vi "DAQAdvance.vi"() -> ()   [LabVIEW 2018]
uses:
  <vilib>/DAQmx/read.llb/DAQmx Read (Analog DBL 1Chan 1Samp).vi
  <vilib>/DAQmx/write.llb/DAQmx Write (Analog DBL 1Chan 1Samp).vi
  <vilib>/DAQmx/miscellaneous.llb/DAQmx Fill In Error Info.vi
panel:
  out "Waveform Chart":cluster{dbl, "data":dbl}(graph)
  in  "y":i32
  in  "stop":bool
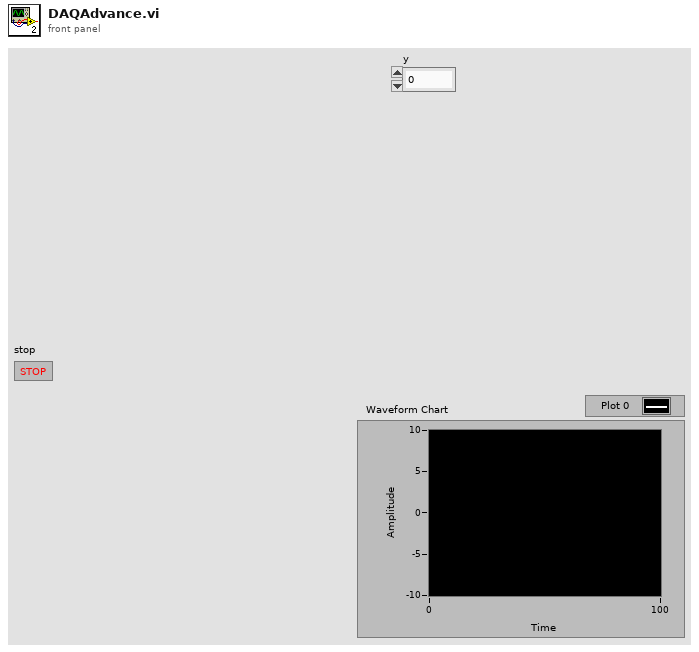
[diagram p1: front panel]
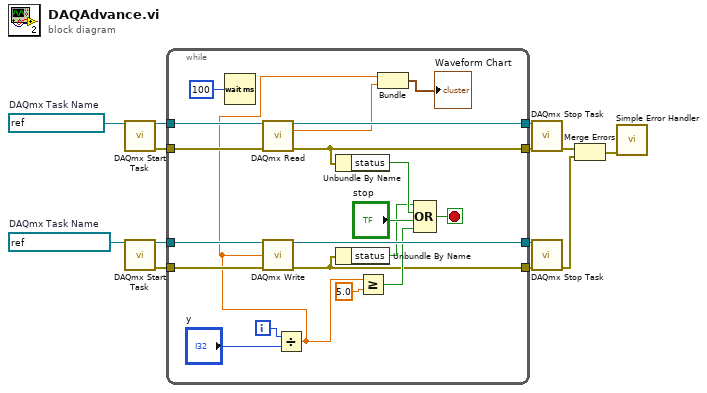
[diagram p0: block diagram]
diagram:
  w6 = refnum<k21> "DAC-valjund0"  # DAQmx Task Name
  w9 = refnum<k21> "ADC-sisend0"  # DAQmx Task Name
  n1 = call <vilib>:"DAQmx Start Task.vi"("task/channels in"=w9) -> ("task out"=w11:refnum<k21>, "error out"=w13:errorcluster)  [unwired: 13 in]
  n2 = call <vilib>:"DAQmx Start Task.vi"("task/channels in"=w6) -> ("task out"=w7:refnum<k21>, "error out"=w8:errorcluster)  [unwired: 13 in]
  n3 = while {
    tunnel: w13 -> [w32]
    tunnel: [w30] -> w12
    tunnel: w11 -> [w31]
    tunnel: [w29] -> w10
    tunnel: w8 -> [w28]
    tunnel: w7 -> [w27]
    tunnel: [w26] -> w5
    tunnel: [w17] -> w4
    i -> [w25]
    stop <- w20 stop-if-true
    n4 = Wait (ms)(milliseconds to wait=u32 100) -> ()  [unwired: 1 out]
    n5 = call-poly <vilib>:"DAQmx Read.vi"("task/channels in"=w31, "error in"=w32) -> ("task out"=w29:refnum<k21>, "data"=w16:dbl, "error out"=w30:errorcluster)  [unwired: 11 in]
    n6 = Divide(x=w25, y="y") -> (x/y=w15:dbl)
    n7 = call-poly <vilib>:"DAQmx Write.vi"("task/channels in"=w27, "data"=w15, "error in"=w28) -> ("task out"=w26:refnum<k21>, "error out"=w17:errorcluster)  [unwired: 10 in, 1 out]
    n8 = Unbundle By Name(w30) -> ("status"=w19:bool)
    n9 = Unbundle By Name(w17) -> ("status"=w18:bool)
    n10 = Greater Or Equal?(x=w15, y=5.0) -> (x >= y?=w21:bool)
    n11 = Bundle(w15, "data"=w16) -> (→"Waveform Chart":cluster{dbl, "data":dbl})  [unwired: 1 in]
    n12 = Compound Arithmetic op=OR(w18, w19, "stop", w21) -> (w20:bool)
  }
  n13 = call <vilib>:"DAQmx Stop Task.vi"("task/channels in"=w10, "error in"=w12) -> ("error out"=w3:errorcluster)  [unwired: 12 in, 1 out]
  n14 = call <vilib>:"DAQmx Stop Task.vi"("task/channels in"=w5, "error in"=w4) -> ("error out"=w2:errorcluster)  [unwired: 12 in, 1 out]
  n15 = Merge Errors(w3, w2) -> (w1:errorcluster)
  n16 = call <vilib>:"Simple Error Handler.vi"("error in (no error)"=w1) -> ()  [unwired: 4 in, 5 out]
